vi "Process_Run With Elevation.vi"(8 "error in (no error)":errorcluster, 11 "fileName":path=path "C:/Users/Phalanx/Desktop/Exemples 1/TestScript.bat") -> (0 "error out":errorcluster)   [LabVIEW 2021]
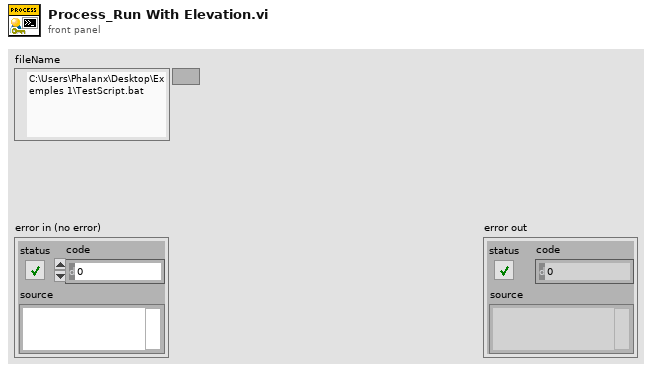
[diagram p1: front panel]
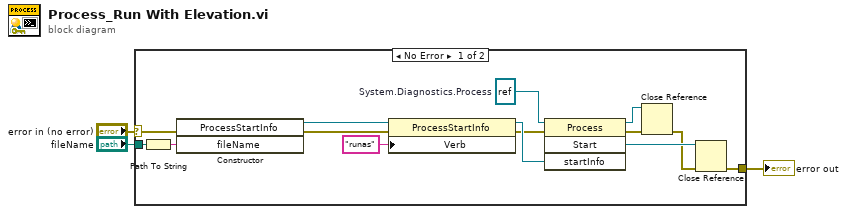
[diagram p0: block diagram]
diagram:
  n1 = case shown="No Error" "error in (no error)" {
    selector: "error in (no error)" -> [w8 w18]
    tunnel: "fileName" -> [w9 _]
    tunnel: [w7 w18] -> w1
    frame No Error {
      w17 = refnum<k24> refnum  # System.Diagnostics.Process
      n2 = Path To String(path=w9) -> (string=w4:string)
      n3 = constructor class="ProcessStartInfo"(error in=w8, "fileName"=w4) -> (reference out=w16:refnum<k24>, error out=w12:errorcluster)  [unwired: 2 in, 2 out]
      n4 = property class="ProcessStartInfo"(reference=w16, error in=w12, "Verb"="runas") -> (reference out=w15:refnum<k24>, error out=w13:errorcluster)
      n5 = invoke class="Process" method="Start"(reference=w17, error in=w13, "startInfo"=w15) -> (reference out=w11:refnum<k24>, error out=w10:errorcluster, "Start"=w6:refnum<k24>)  [unwired: 1 in, 1 out]
      n6 = Close Reference(reference=w11, error in (no error)=w10) -> (error out=w5:errorcluster)
      n7 = Close Reference(reference=w6, error in (no error)=w5) -> (error out=w7:errorcluster)
    }
    frame Error {
    }
  }
  "error out" <- w1
